vi "TektronixMDO_Readout_writeFile.vi"() -> ()   [LabVIEW 2016]
doc: "This example illustrates how to use autosetup and continuously acquires waveforms from a single channel using the following steps:\n\n1. Specify a valid VISA session. \n2. Specify a channel. \n3. Specify a time-out value for reading waveform.\n4. Run the VI. The graph displays the waveform you acquire."
uses:
  <instrlib>/Tektronix DPO MSO 2000 4000 Series/Public/Configure/Configure Trigger (Edge).vi
  <instrlib>/Tektronix DPO MSO 2000 4000 Series/Public/Data/Read (Single Waveform).vi
  <instrlib>/Tektronix DPO MSO 2000 4000 Series/Tektronix DPO MSO 2000 4000 Series.lvlib
panel:
  out "Event":i32
  in  "Target total event":i32
  out "dt":dbl format="%#_13g"
  out "Histogram":dynamicdata(graph)
  in  "Operator":string="Hsin-Yeh"
  in  "file path":path=path "C:/Users/NTU/Desktop/Chih-Ping/NaI0827/1-haveNumber/Co60/Co60_5.tdms"
  in  "Timebase (0.0005 s)":dbl=0.0005
  in  "Position (10 %)":dbl=10.0
  in  "Record Length (10: 10k points)":u32(ring)=10 items=["1000 points"=1, "10k points"=10, "100k points"=100, "1M points"=1000, "5M points"=5000, "10M points"=10000]
  in  "Trigger Slope (0: Rising)":u16(ring) items=["Rising", "Falling", "Either"]
  in  "Trigger Level (0.0 V)":dbl
  in  "Trigger Source (0: Channel 1)":u16(ring) items=["Channel 1", "Channel 2", "Channel 3", "Channel 4", "AC Line", "Aux", "Digital Channel 0", "Digital Channel 1", "Digital Channel 2", "Digital Channel 3", "Digital Channel 4", "Digital Channel 5", "Digital Channel 6", "Digital Channel 7", "Digital Channel 8", "Digital Channel 9", "Digital Channel 10", "Digital Channel 11", "Digital Channel 12", "Digital Channel 13", "Digital Channel 14", "Digital Channel 15", "RF"]
  in  "Trigger Coupling (0 : DC)":u16(ring) items=["DC", "HF Reject", "LF Reject", "Noise Reject", "AC"]
  in  "Bandwidth (0: FULL)":u16(ring) items=["FULL", "250 MHz", "150 MHz", "20 MHz"]
  in  "Vertical Offset (0.0 V)":dbl
  in  "Vertical Range (10.0 V)":dbl=10.0
  in  "Probe Attenuation (1)":dbl=1.0
  in  "Vertical Coupling (1: DC)":u16(ring)=1 items=["AC", "DC", "Ground", "DC Reject"]
  in  "Channel (0: Channel 1) 2":u16(ring) items=["Channel 1", "Channel 2", "Channel 3", "Channel 4", "Math", "Reference 1", "Reference 2", "Reference 3", "Reference 4", "Bus 1", "Bus 2"]
  in  "Input Impedance (0: 1M ohm)":u16(ring) items=["1M", "75", "50"]
  in  "Enable Channel (T: Enable)":bool=TRUE
  in  "Channel (0: Channel 1)":u16(ring) items=["Channel 1", "Channel 2", "Channel 3", "Channel 4", "Math", "Reference 1", "Reference 2", "Reference 3", "Reference 4"]
  in  "Maximum Time (10000ms)":u32=10000
  in  "stop":bool
  in  "VISA Resource Name":refnum<visa-resource-name>
  out "Waveform Graph":waveform(dbl)(graph)
  # "(C) 2006 - 2022. National Instruments Corporation. ALL RIGHTS RESERVED."
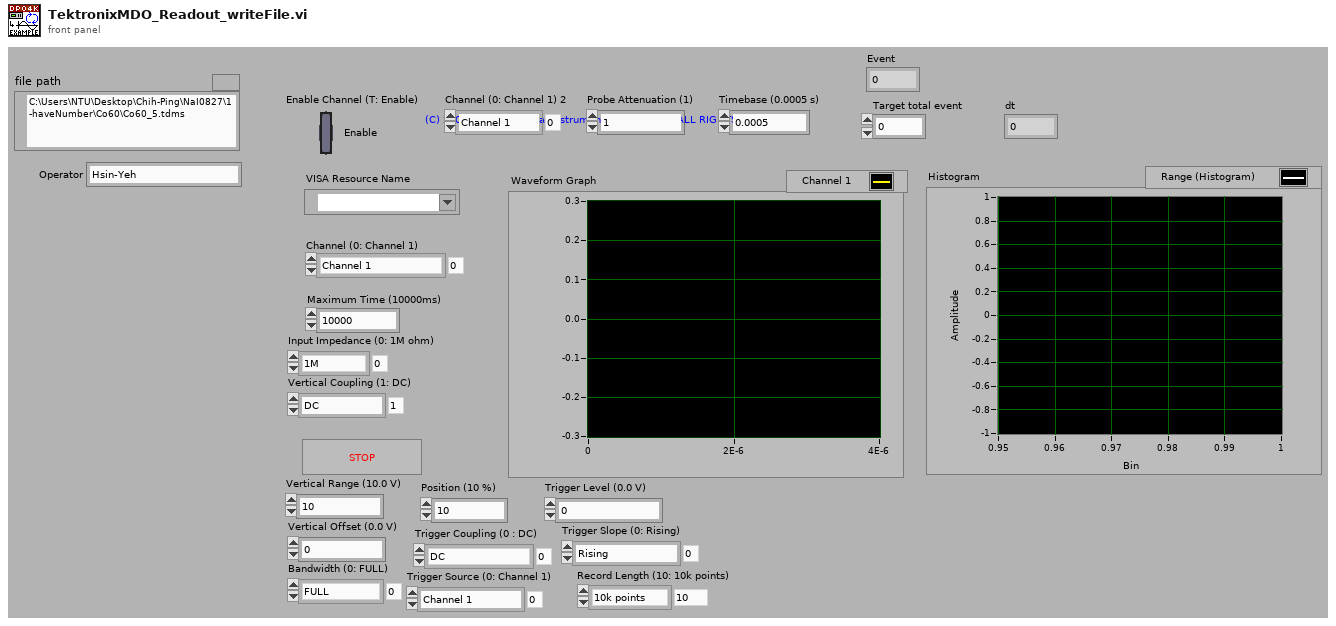
[diagram p1: front panel]
types:
  T1 = enum16{"open", "open or create", "create or replace", "create", "open (read-only)"}
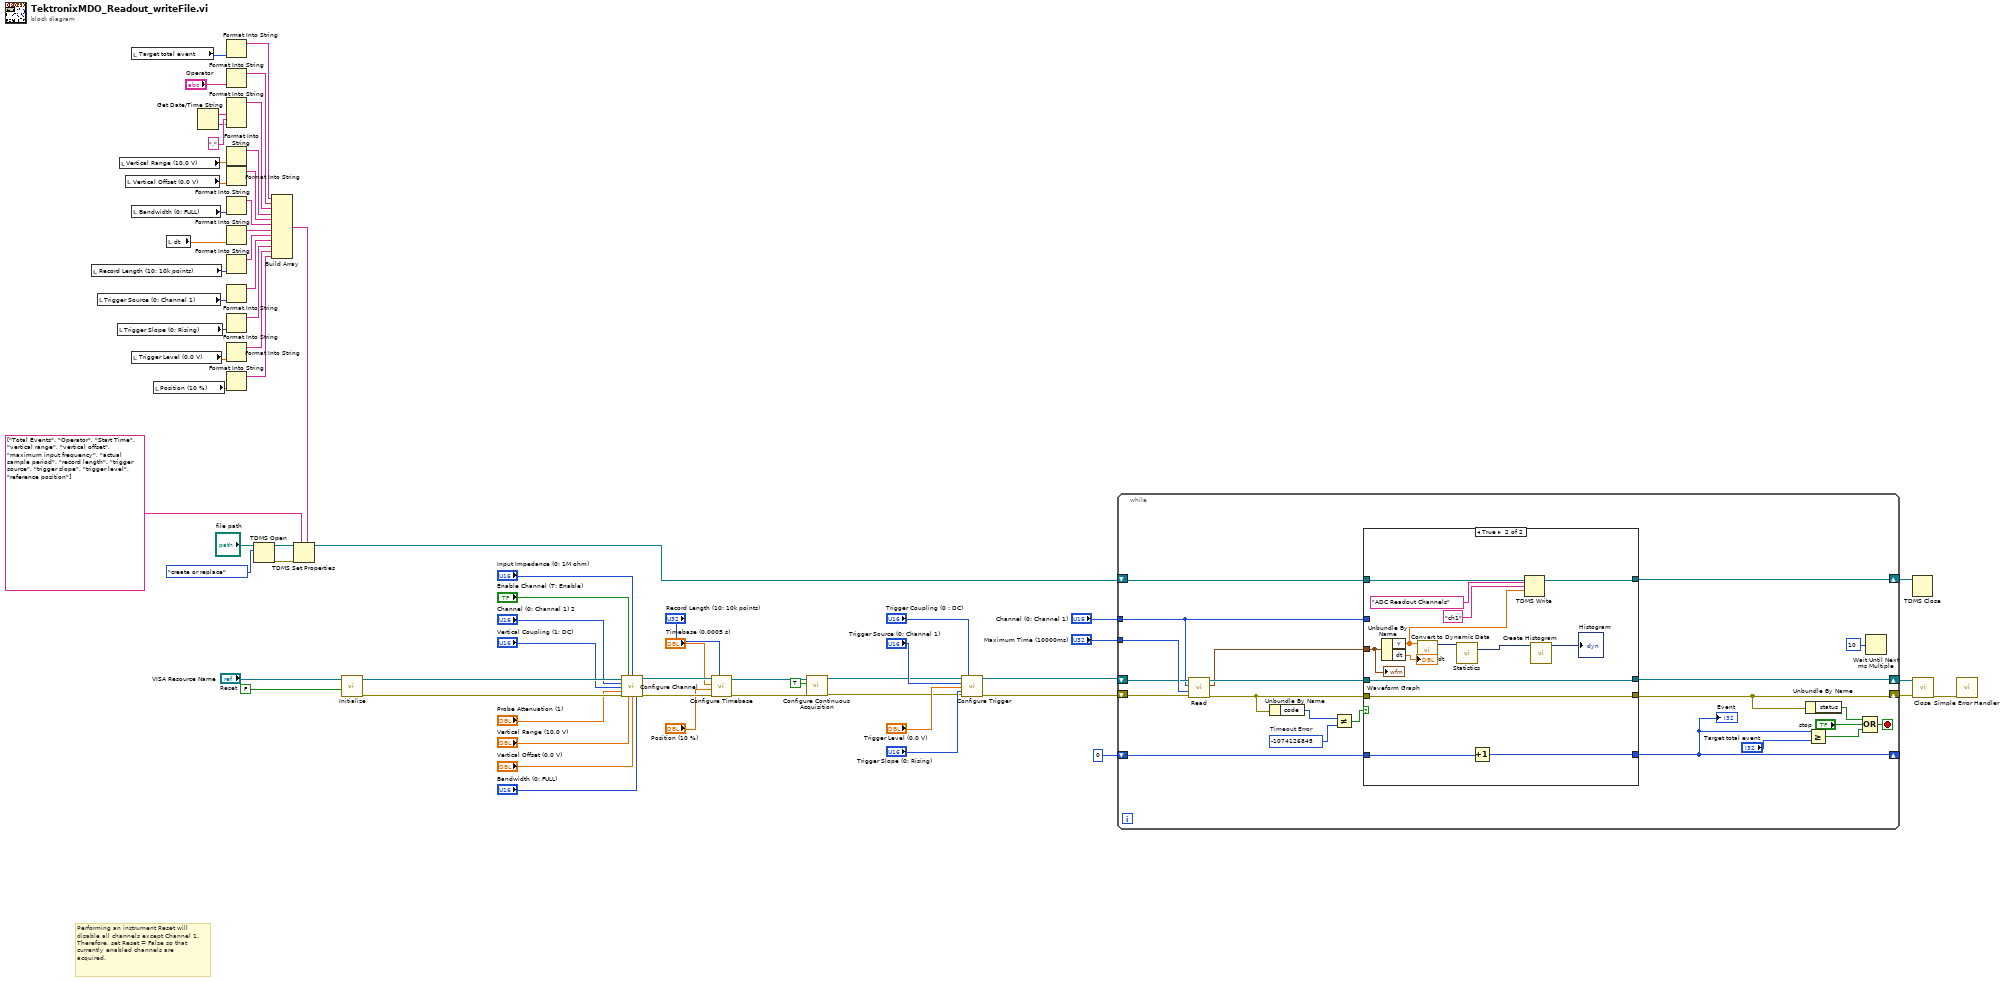
[diagram p0: block diagram]
diagram:
  w65 = FALSE  # Reset
  # "Performing an instrument Reset will disable all channels except Channel 1. Therefore, set Reset = False so that currently enabled channels are acquired."
  n1 = local read "Record Length (10: 10k points)"() -> (w37:u32)
  n2 = local read "Trigger Source (0: Channel 1)"() -> (w36:u16)
  n3 = local read "Trigger Slope (0: Rising)"() -> (w23:u16)
  n4 = local read "Vertical Range (10.0 V)"() -> (w35:dbl)
  n5 = local read "Vertical Offset (0.0 V)"() -> (w32:dbl)
  n6 = local read "Target total event"() -> (w11:i32)
  n7 = local read "Bandwidth (0: FULL)"() -> (w31:u16)
  n8 = local read "Trigger Level (0.0 V)"() -> (w38:dbl)
  n9 = local read "Position (10 %)"() -> (w33:dbl)
  n10 = local read "dt"() -> (w34:dbl)
  n11 = Get Date/Time String() -> (date string=w29:string, time string=w27:string)  [unwired: 3 in]
  n12 = Format Into String(w11) -> (resulting string=w39:string)  [unwired: 3 in, 1 out]
  n13 = Format Into String("Operator") -> (resulting string=w26:string)  [unwired: 3 in, 1 out]
  n14 = Format Into String(w29, "," ("input 2"), w27) -> (resulting string=w25:string)  [unwired: 3 in, 1 out]
  n15 = Format Into String(w35) -> (resulting string=w24:string)  [unwired: 3 in, 1 out]
  n16 = Format Into String(w32) -> (resulting string=w21:string)  [unwired: 3 in, 1 out]
  n17 = Format Into String(w31) -> (resulting string=w22:string)  [unwired: 3 in, 1 out]
  n18 = Format Into String(w34) -> (resulting string=w20:string)  [unwired: 3 in, 1 out]
  n19 = Format Into String(w37) -> (resulting string=w19:string)  [unwired: 3 in, 1 out]
  n20 = Format Into String(w36) -> (resulting string=w18:string)  [unwired: 3 in, 1 out]
  n21 = Format Into String(w23) -> (resulting string=w17:string)  [unwired: 3 in, 1 out]
  n22 = Format Into String(w38) -> (resulting string=w16:string)  [unwired: 3 in, 1 out]
  n23 = Format Into String(w33) -> (resulting string=w15:string)  [unwired: 3 in, 1 out]
  n24 = TDMS Open(10:T1."create or replace" ("operation (0:open)"), 11:"file path") -> (0:w41:errorcluster, 3:w40:refnum<k34>)  [unwired: 5 in]
  n25 = Build Array(w39, w26, w25, w24, w21, w22, w20, w19, w18, w17, w16, w15) -> (w14:string[])
  n26 = TDMS Set Properties(5:w14, 7:string[] ["Total Events", "Operator", "Start Time", "vertical range", "vertical offset", "maximum input frequency", "actual sample period", "record length", "trigger source", "trigger slope", "trigger level", "reference position"], 8:w41, 11:w40) -> (3:w10:refnum<k34>)  [unwired: 2 in, 3 out]
  n27 = call <instrlib>:"Initialize.vi"("Reset (True)"=w65, "VISA resource name"="VISA Resource Name") -> ("error out"=w61:errorcluster, "VISA resource name out"=w62:refnum<visa-resource-name>)  [unwired: 8 in]
  n28 = call <instrlib>:"Configure Channel.vi"("VISA resource name"=w62, "Enable Channel (T: Enable)"="Enable Channel (T: Enable)", "Input Impedance (0: 1M ohm)"="Input Impedance (0: 1M ohm)", "Channel (0: Channel 1)"="Channel (0: Channel 1) 2", "Vertical Coupling (1: DC)"="Vertical Coupling (1: DC)", "Probe Attenuation (1)"="Probe Attenuation (1)", "error in (no error)"=w61, "Vertical Range (10.0 V)"="Vertical Range (10.0 V)", "Vertical Offset (0.0 V)"="Vertical Offset (0.0 V)", "Bandwidth (0: FULL)"="Bandwidth (0: FULL)") -> ("VISA resource name out"=w48:refnum<visa-resource-name>, "error out"=w47:errorcluster)  [unwired: 4 in]
  n29 = call <instrlib>:"Configure Timebase.vi"("Record Length (10: 10k points)"="Record Length (10: 10k points)", "error in (no error)"=w47, "Position (10 %)"="Position (10 %)", "Timebase (0.0005 s)"="Timebase (0.0005 s)", "VISA resource name"=w48) -> ("error out"=w3:errorcluster, "VISA resource name out"=w5:refnum<visa-resource-name>)  [unwired: 5 in]
  n30 = call <instrlib>:"Configure Continuous Acquisition.vi"("error in (no error)"=w3, "Enable Continuous Acquisition Mode (T: Enable)"=TRUE, "VISA resource name"=w5) -> ("error out"=w2:errorcluster, "VISA resource name out"=w4:refnum<visa-resource-name>)  [unwired: 7 in]
  n31 = call-poly <instrlib>:"Configure Trigger.vi"("VISA resource name"=w4, "Trigger Coupling (0 : DC)"="Trigger Coupling (0 : DC)", "Trigger Source (0: Channel 1)"="Trigger Source (0: Channel 1)", "Trigger Level (0.0 V)"="Trigger Level (0.0 V)", "Trigger Slope (0: Rising)"="Trigger Slope (0: Rising)", "error in (no error)"=w2) -> ("VISA resource name out"=w13:refnum<visa-resource-name>, "error out"=w7:errorcluster)  [unwired: 8 in]
  n32 = while {
    tunnel: "Maximum Time (10000ms)" -> [w88]
    tunnel: "Channel (0: Channel 1)" -> [w84]
    shift-right: [w85] -> w67
    shift-left: w13 -> [w87]
    shift-right: [w73] -> w8
    shift-left: w10 -> [w74]
    shift-right: [w69] -> _
    shift-left: 0 -> [w80]
    shift-right: [w71] -> w6
    shift-left: w7 -> [w72]
    stop <- w75 stop-if-true
    w82 = -1074126845  # Timeout Error
    n33 = call-poly <instrlib>:"Read.vi"("error in (no error)"=w72, "Maximum Time (10000ms)"=w88, "Channel (0: Channel 1)"=w84, "VISA resource name"=w87) -> ("error out"=w71:errorcluster, "Waveform Graph"=w70:waveform(dbl), "VISA resource name out"=w86:refnum<visa-resource-name>)  [unwired: 5 in]
    n34 = Unbundle By Name(w71) -> ("code"=w83:i32)
    n35 = Not Equal?(x=w83, y=w82) -> (x != y?=w81:bool)
    n36 = case shown="True" w81 {
      tunnel: w86 -> [w93 w101]
      tunnel: [w93 w101] -> w85
      tunnel: w71 -> [w92 w97]
      tunnel: [w92 w97] -> _
      tunnel: w84 -> [_ _]
      tunnel: w80 -> [w91 w106]
      tunnel: [w91 w105] -> w69
      tunnel: w74 -> [w90 w104]
      tunnel: [w90 w102] -> w73
      tunnel: w70 -> [_ w96]
      frame False {
      }
      frame True {
        n37 = Unbundle By Name(w96) -> ("Y"=w99:dbl[], "dt"=→"dt":dbl)
        n38 = call "Convert to Dynamic Data"("Array"=w99) -> ("Dynamic Data Type"=w100:dynamicdata)  [unwired: 3 in]
        n39 = call "Statistics"("Signals"=w100) -> ("Range"=w95:dynamicdata)  [unwired: 25 in, 1 out]
        n40 = Increment(x=w106) -> (x+1=w105:i32)
        n41 = TDMS Write(0:w104, 5:"ADC Readout Channels" ("group name (Untitled)"), 7:"ch1", 9:w99) -> (4:w102:refnum<k34>)  [unwired: 2 in, 3 out]
        n42 = call "Create Histogram"("Signal"=w95) -> ("Histogram"=→"Histogram":dynamicdata)  [unwired: 9 in, 1 out]
        "Waveform Graph" <- w96
      }
    }
    "Event" <- w69
    n43 = Unbundle By Name(w71) -> ("status"=w78:bool)
    n44 = Greater Or Equal?(x=w69, y="Target total event") -> (x >= y?=w76:bool)
    n45 = Compound Arithmetic op=OR(w78, "stop", w76) -> (w75:bool)
    n46 = Wait Until Next ms Multiple(millisecond multiple=u32 10) -> ()  [unwired: 1 out]
  }
  n47 = TDMS Close(11:w8) -> ()  [unwired: 1 in, 2 out]
  n48 = call <instrlib>:"Close.vi"("error in (no error)"=w6, "VISA resource name"=w67) -> ("error out"=w66:errorcluster)  [unwired: 9 in]
  n49 = call <vilib>:"Simple Error Handler.vi"("error in (no error)"=w66) -> ()  [unwired: 4 in, 5 out]
